vi "Read Sizes.vi"(8 "error in (no error)":errorcluster, 11 "TG Base Graph in":refnum<class "Base Graph.lvclass">) -> (0 "error out":errorcluster, 2 "Sizes":cluster{"Height":u32, "Width":u32}, 3 "TG Base Graph out":refnum<class "Base Graph.lvclass">)   [LabVIEW 2023, in "Base Graph.lvclass"]
uses:
  Base Graph.lvclass
  Base Graph.lvclass/Base Graph.ctl
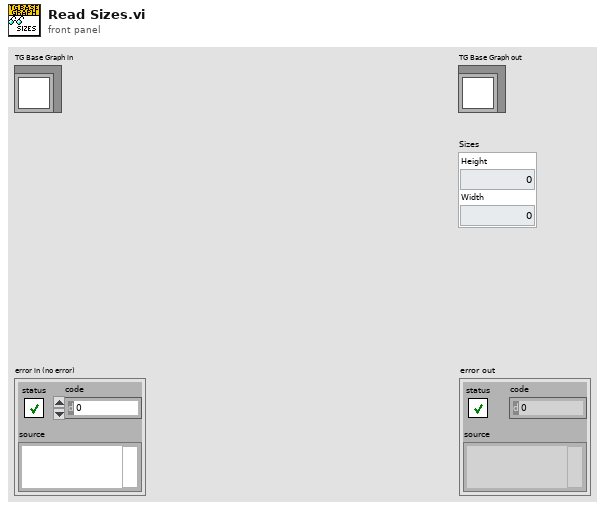
[diagram p1: front panel]
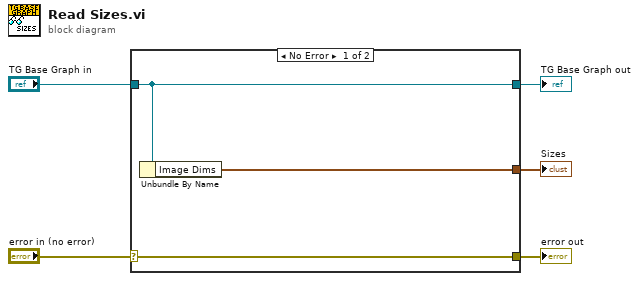
[diagram p0: block diagram]
diagram:
  n1 = case shown="No Error" "error in (no error)" {
    selector: "error in (no error)" -> [w8 w9]
    tunnel: [w8 w9] -> w4
    tunnel: [w7 w10] -> w2
    tunnel: "TG Base Graph in" -> [w7 w10]
    tunnel: [w6 _] -> w1
    frame No Error {
      n2 = Unbundle By Name(w7) -> ("Image Dims"=w6:cluster{"Height":u32, "Width":u32})
    }
    frame Error {
    }
  }
  "error out" <- w4
  "TG Base Graph out" <- w2
  "Sizes" <- w1
